vi "Dictionary Test - 003.vi"(8 "error in (no error)":errorcluster) -> (0 "error out":errorcluster, 2 "pass":bool)   [LabVIEW 2009]
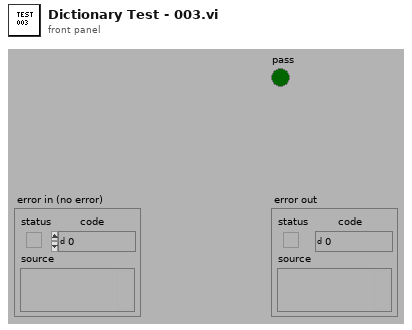
[diagram p1: front panel]
types:
  T1 = typedef "Dictionary Object RefNum.ctl" = refnum<k1>
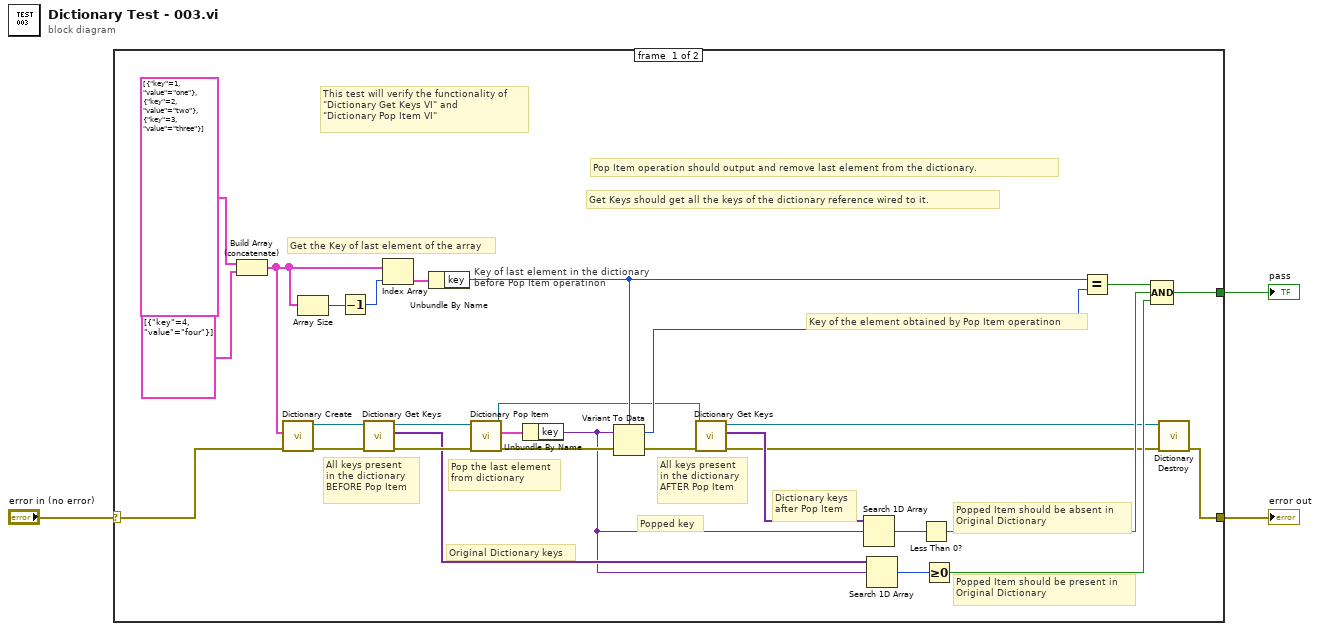
[diagram p0: block diagram]
diagram:
  n1 = case shown="No Error" "error in (no error)" {
    selector: "error in (no error)" -> [w32 w33]
    tunnel: [w31 w33] -> w1
    tunnel: [w6 _] -> w3
    frame #0 {
      # "Get Keys should get all the keys of the dictionary reference wired to it."
      # "Pop Item operation should output and remove last element from the dictionary."
      # "Dictionary keys\nafter Pop Item"
      # "Popped key"
      # "Original Dictionary keys"
      # "Popped Item should be present in\nOriginal Dictionary"
      # "Popped Item should be absent in\nOriginal Dictionary"
      # "All keys present \nin the dictionary\nAFTER Pop Item"
      # "Key of the element obtained by Pop Item operatinon"
      # "Key of last element in the dictionary\nbefore Pop Item operatinon"
      # "Pop the last element\nfrom dictionary"
      # "All keys present \nin the dictionary\nBEFORE Pop Item"
      # "Get the Key of last element of the array"
      # "This test will verify the functionality of \n\"Dictionary Get Keys VI\" and \n\"Dictionary Pop Item VI\""
      n2 = Build Array (concatenate)(cluster{"key":i32, "value":string}[] [{"key"=1, "value"="one"}, {"key"=2, "value"="two"}, {"key"=3, "value"="three"}] ("dictionary with updates"), cluster{"key":i32, "value":string}[] [{"key"=4, "value"="four"}] ("initial dictionary (empty)")) -> (w19:cluster{"key":i32, "value":string}[])
      n3 = call "Dictionary Create.vi"("error in (no error)"=w32, "initial dictionary (empty)"=w19) -> ("error out"=w25:errorcluster, "dictionary out"=w28:T1)  [unwired: 8 in]
      n4 = Array Size(array=w19) -> (size(s)=w18:i32)
      n5 = Decrement(x=w18) -> (x-1=w17:i32)
      n6 = call "Dictionary Get Keys.vi"("error in (no error)"=w25, "dictionary"=w28) -> ("error out"=w27:errorcluster, "keys"=w14:variant[], "dictionary out"=w20:T1)  [unwired: 7 in]
      n7 = Index Array(array=w19, index=w17) -> (element=w23:cluster{"key":i32, "value":string})
      n8 = Unbundle By Name(w23) -> ("key"=w22:i32)
      n9 = call "Dictionary Pop Item.vi"("error in (no error)"=w27, "dictionary"=w20) -> ("error out"=w26:errorcluster, "item"=w24:cluster{"key":variant, "value":variant}, "dictionary out"=w15:T1)  [unwired: 7 in]
      n10 = Unbundle By Name(w24) -> ("key"=w10:variant)
      n11 = Variant To Data(error in=w26, Variant=w10, type=w22) -> (error out=w16:errorcluster, data=w21:i32)
      n12 = call "Dictionary Get Keys.vi"("error in (no error)"=w16, "dictionary"=w15) -> ("error out"=w5:errorcluster, "keys"=w11:variant[], "dictionary out"=w4:T1)  [unwired: 7 in]
      n13 = Search 1D Array(1D array=w11, element=w10) -> (index of element=w12:i32)  [unwired: 1 in]
      n14 = Search 1D Array(1D array=w14, element=w10) -> (index of element=w13:i32)  [unwired: 1 in]
      n15 = Less Than 0?(x=w12) -> (x < 0?=w9:bool)
      n16 = Greater Or Equal To 0?(x=w13) -> (x >= 0?=w8:bool)
      n17 = Equal?(x=w22, y=w21) -> (x = y?=w7:bool)
      n18 = Compound Arithmetic op=AND(w7, w9, w8) -> (w6:bool)
      n19 = call "Dictionary Destroy.vi"("error in (no error)"=w5, "dictionary"=w4) -> ("error out"=w31:errorcluster)  [unwired: 9 in]
    }
    frame #1 {
    }
  }
  "pass" <- w3
  "error out" <- w1
